vi "DLL Download.vi"(1 "Pre-Release?":bool, 2 "Overwrite":bool, 11 "Error In":errorcluster) -> (15 "Error Out":errorcluster)   [LabVIEW 2013, in "GEA2_Toolkit.lvlib"]
uses:
  library/GEA2_Toolkit.lvlib
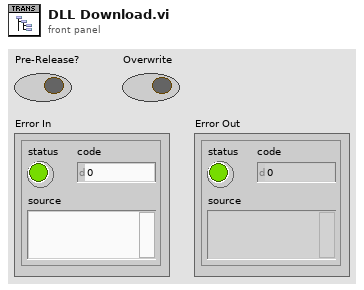
[diagram p1: front panel]
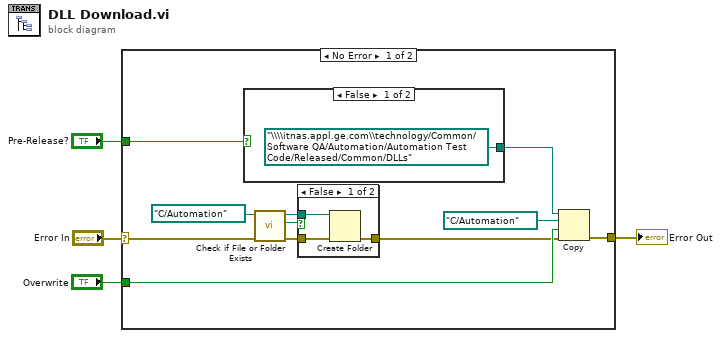
[diagram p0: block diagram]
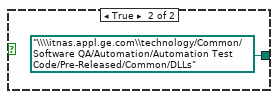
[diagram p3: hidden frame]
diagram:
  n1 = case shown="No Error" "Error In" {
    selector: "Error In" -> [w12 w22]
    tunnel: "Pre-Release?" -> [w13 _]
    tunnel: [w5 w22] -> w3
    tunnel: "Overwrite" -> [w14 _]
    frame No Error {
      n2 = case shown="False" w13 {
        tunnel: [path "\\\\itnas.appl.ge.com\\technology/Common/Software QA/Automation/Automation Test Code/Released/Common/DLLs" ("Product Source Path 2") path "\\\\itnas.appl.ge.com\\technology/Common/Software QA/Automation/Automation Test Code/Pre-Released/Common/DLLs" ("Product Source Path 2")] -> w15
        frame False {
        }
        frame True {
        }
      }
      n3 = call <vilib>:"Check if File or Folder Exists.vi"("error in (no error)"=w12, "path"=path "C:/Automation" ("target path (use dialog)")) -> ("error out"=w10:errorcluster, "file or folder exists?"=w11:bool, "dup path"=w9:path)  [unwired: 7 in]
      n4 = case shown="False" w11 {
        tunnel: w10 -> [w18 w19]
        tunnel: w9 -> [w17 _]
        tunnel: [w16 w19] -> w8
        frame False {
          n5 = Create Folder(path (use dialog)=w17, error in=w18) -> (error out=w16:errorcluster)  [unwired: 1 in, 2 out]
        }
        frame True {
        }
      }
      n6 = Copy(8:w8, 9:w14, 10:path "C:/Automation" ("target path (use dialog)"), 11:w15) -> (0:w5:errorcluster)  [unwired: 1 in, 2 out]
    }
    frame Error {
    }
  }
  "Error Out" <- w3
